vi "CONEXION_V1.vi"() -> ()   [LabVIEW 2021]
panel:
  out "CABINA A":dbl(slide) scale=1.0..5.0
  in  "BAJA B":bool
  in  "SUBE B":bool
  in  "SUBE A":bool
  in  "BAJA A":bool
  in  "stop":bool
  in  "FS A 1":bool
  out "LUZ VERDE":bool
  out "LUZ ROJA":bool
  out "RELE SUB B":bool
  out "MOTOR B":bool
  out "RELE SUB A":bool
  out "MOTOR A":bool
  in  "PPB 5":bool
  in  "PPB 4":bool
  in  "PPB 3":bool
  in  "PPB 2":bool
  in  "PPB 1":bool
  in  "PPA 5":bool
  in  "PPA 4":bool
  in  "PPA 3":bool
  in  "PPA 2":bool
  in  "PPA 1":bool
  in  "DEMOSTRATIVA":bool
  in  "COLECTIVA":bool
  in  "UNIVERSAL":bool
  in  "FS B 5":bool
  in  "FS B 4":bool
  in  "FS B 3":bool
  in  "FS B 2":bool
  in  "FS B 1":bool
  in  "FS A 5":bool
  in  "FS A 4":bool
  in  "FS A 3":bool
  in  "FS A 2":bool
  in  "STOP":bool
  in  "START":bool
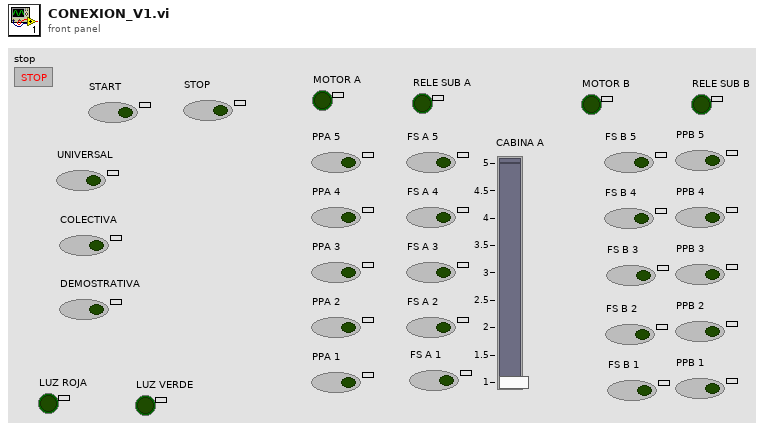
[diagram p1: front panel]
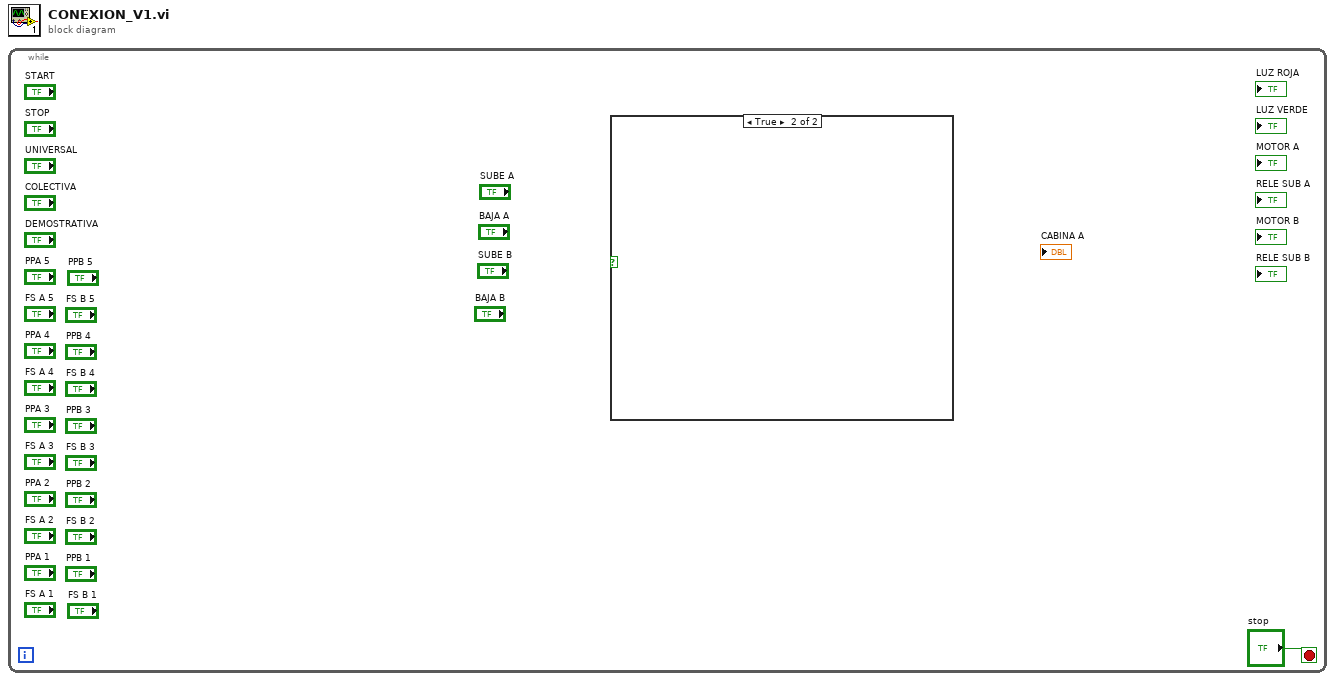
[diagram p0: block diagram]
diagram:
  n1 = while {
    stop <- "stop" stop-if-true
    n2 = case shown="True" {
      selector: _ -> [_ _]
      frame False {
      }
      frame True {
      }
    }
  }
